vi "PositionControl.vi"(6 "ConsecutiveTargets":i32, 7 "ErrorDeadband":dbl, 8 "MaxOutput":dbl, 9 "MinOutput":dbl, 10 "ErrorThreshold":dbl, 11 "Error":dbl) -> (0 "UnfilteredOnTarget":bool, 2 "OnTarget":bool, 3 "OutputValue":dbl)   [LabVIEW 2023]
doc: "Calculates an output to help reach a target based on the current error and calibration parameters.\n\nInputs:\n-- ErrorDeadband -- Double -- The Deadband or range of values that will be considered to be \"ontarget\" --\n-- Error -- Double -- The Error of your current value from the target value (Target - Value) --\n-- MinOutput -- Double -- The minimum output the system is capable of outputting -- \n-- MaxOutput -- Double -- The maximum output the system is capableof outputting-\n-- ConsecutiveTargets -- Boolean -- The number of times you must remain on target to confidently be on target --\n\nOutputs:\n-- OutputValue -- Double -- The output value desired to help reach your target --\n-- OnTarget -- Boolean -- True if you are confidently on target --\n-- UnfilteredOnTarget -- Boolean -- True if position control thinks you are on target for 1 loop. NOT RECOMENDED FOR USE IN ROBOT CODE, only meant for debugging --"
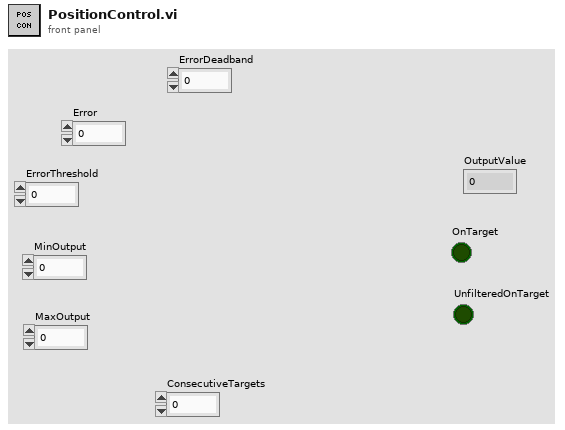
[diagram p1: front panel]
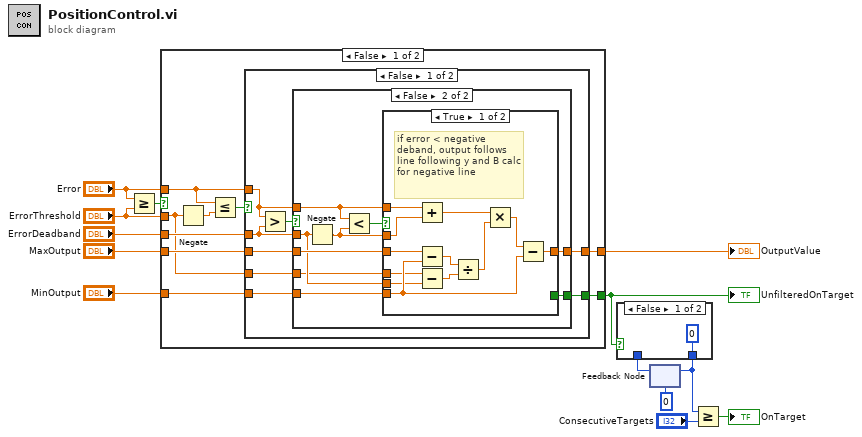
[diagram p0: block diagram]
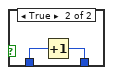
[diagram p2: hidden frame]
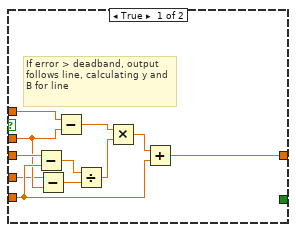
[diagram p3: hidden frame]
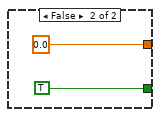
[diagram p4: hidden frame]
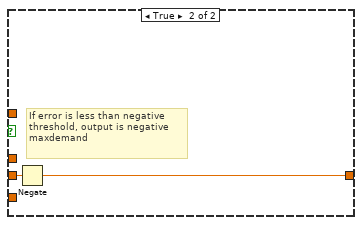
[diagram p5: hidden frame]
diagram:
  n1 = Greater Or Equal?(x="Error", y="ErrorThreshold") -> (x >= y?=w11:bool)
  n2 = case shown="False" w11 {
    tunnel: [w19 w67] -> w13
    tunnel: "MaxOutput" -> [w20 w67]
    tunnel: "Error" -> [w18 _]
    tunnel: "ErrorThreshold" -> [w14 _]
    tunnel: "ErrorDeadband" -> [w17 _]
    tunnel: "MinOutput" -> [w16 _]
    tunnel: [w15 _] -> w3
    frame False {
      n3 = Negate(x=w14) -> (-x=w21:dbl)
      n4 = Less Or Equal?(x=w18, y=w21) -> (x <= y?=w22:bool)
      n5 = case shown="False" w22 {
        tunnel: w20 -> [w25 w66]
        tunnel: [w29 w65] -> w19
        tunnel: w18 -> [w27 _]
        tunnel: w17 -> [w26 _]
        tunnel: w16 -> [w28 _]
        tunnel: [w24 _] -> w15
        tunnel: w14 -> [w23 _]
        frame False {
          n6 = Greater?(x=w27, y=w26) -> (0:w30:bool)
          n7 = case shown="False" w30 {
            tunnel: [w41 w50] -> w29
            tunnel: w28 -> [w34 w46]
            tunnel: w27 -> [w40 w48]
            tunnel: w26 -> [w32 w43]
            tunnel: w25 -> [w35 w47]
            tunnel: [_ w45] -> w24
            tunnel: w23 -> [w31 w42]
            frame True {
              # "If error > deadband, output follows line, calculating y and B for line"
              n8 = Subtract(x=w35, y=w34) -> (x-y=w37:dbl)
              n9 = Subtract(x=w31, y=w32) -> (x-y=w36:dbl)
              n10 = Subtract(x=w40, y=w32) -> (x-y=w39:dbl)
              n11 = Divide(x=w37, y=w36) -> (x/y=w38:dbl)
              n12 = Multiply(x=w39, y=w38) -> (x*y=w33:dbl)
              n13 = Add(x=w33, y=w34) -> (x+y=w41:dbl)
            }
            frame False {
              n14 = Negate(x=w43) -> (-x=w44:dbl)
              n15 = Less?(x=w48, y=w44) -> (x < y?=w49:bool)
              n16 = case shown="True" w49 {
                tunnel: [w62 0.0] -> w50
                tunnel: w46 -> [w54 _]
                tunnel: w48 -> [w61 _]
                tunnel: w44 -> [w60 _]
                tunnel: w47 -> [w55 _]
                tunnel: [_ TRUE] -> w45
                tunnel: w43 -> [w52 _]
                tunnel: w42 -> [w51 _]
                frame True {
                  # "if error < negative deband, output follows line following y and B calc for negative line"
                  n17 = Add(x=w61, y=w60) -> (x+y=w59:dbl)
                  n18 = Subtract(x=w55, y=w54) -> (x-y=w57:dbl)
                  n19 = Subtract(x=w51, y=w52) -> (x-y=w56:dbl)
                  n20 = Divide(x=w57, y=w56) -> (x/y=w58:dbl)
                  n21 = Multiply(x=w59, y=w58) -> (x*y=w53:dbl)
                  n22 = Subtract(x=w53, y=w54) -> (x-y=w62:dbl)
                }
                frame False {
                }
              }
            }
          }
        }
        frame True {
          # "If error is less than negative threshold, output is negative maxdemand"
          n23 = Negate(x=w66) -> (-x=w65:dbl)
        }
      }
    }
    frame True {
      # "If error is greater than threshold, output is Maxdemand"
    }
  }
  "OutputValue" <- w13
  "UnfilteredOnTarget" <- w3
  n24 = feedback #1(0) -> (w2:i32)
  n25 = case shown="False" w3 {
    tunnel: w2 -> [_ w70]
    tunnel: [0 w69] -> w1
    frame False {
    }
    frame True {
      n26 = Increment(x=w70) -> (x+1=w69:i32)
    }
  }
  n27 = feedback-in #1(w1) -> ()
  n28 = Greater Or Equal?(x=w1, y="ConsecutiveTargets") -> (x >= y?=→"OnTarget":bool)
